vi "DDPoseEst2_DffDrive_Exec.vi"(8 "error in (no error)":errorcluster) -> (0 "error out":errorcluster)   [LabVIEW 2019]
uses:
  <vilib>/Rock Robotics/WPI/ThirdParty/JAS_Junk/TrajLib/Enum/DIFF_DRIVE_KitBot_WheelSize_ENUM.ctl
  <vilib>/Rock Robotics/WPI/ThirdParty/JAS_Junk/TrajLib/Enum/DIFF_DRIVE_ToughBoxMini_GearChoice_ENUM.ctl
  <vilib>/Rock Robotics/WPI/ThirdParty/JAS_Junk/TrajLib/Enum/DCMOTOR_TYPES_ENUM.ctl
  <vilib>/Rock Robotics/WPI/ThirdParty/JAS_Junk/TrajLib/LinearSystemId_CreateDriveTrainVelocitySystem.vi
  <vilib>/Rock Robotics/WPI/ThirdParty/JAS_Junk/TrajLib/DCMotor_PickMotor.vi
  <vilib>/Rock Robotics/WPI/ThirdParty/JAS_Junk/TrajLib/VI/numCmd_ObtainQueue_TwoDbl.vi
  <vilib>/Rock Robotics/WPI/ThirdParty/JAS_Junk/TrajLib/Units_InchesToMeters.vi
  <vilib>/Rock Robotics/WPI/ThirdParty/JAS_Junk/TrajLib/LinearSystem_New.vi
  <vilib>/Rock Robotics/WPI/ThirdParty/JAS_Junk/TrajLib/MatBuilder_Create.vi
  <vilib>/Rock Robotics/WPI/ThirdParty/JAS_Junk/TrajLib/MatBuilder_Fill.vi
  <vilib>/Rock Robotics/WPI/ThirdParty/JAS_Junk/TrajLib/MatrixHelper_Zero.vi
  <vilib>/Rock Robotics/WPI/ThirdParty/JAS_Junk/TrajLib/DCMotor_GetCIM.vi
  <vilib>/Rock Robotics/WPI/ThirdParty/JAS_Junk/TrajLib/DCMotor_GetAndymark9015.vi
  <vilib>/Rock Robotics/WPI/ThirdParty/JAS_Junk/TrajLib/DCMotor_GetAndymarkRs775_125.vi
  <vilib>/Rock Robotics/WPI/ThirdParty/JAS_Junk/TrajLib/DCMotor_GetBag.vi
  <vilib>/Rock Robotics/WPI/ThirdParty/JAS_Junk/TrajLib/DCMotor_GetBanebotsRs550.vi
  <vilib>/Rock Robotics/WPI/ThirdParty/JAS_Junk/TrajLib/DCMotor_GetBanebotsRs775.vi
  <vilib>/Rock Robotics/WPI/ThirdParty/JAS_Junk/TrajLib/DCMotor_GetFalcon500.vi
  <vilib>/Rock Robotics/WPI/ThirdParty/JAS_Junk/TrajLib/DCMotor_GetMiniCIM.vi
  <vilib>/Rock Robotics/WPI/ThirdParty/JAS_Junk/TrajLib/DCMotor_GetNEO.vi
  <vilib>/Rock Robotics/WPI/ThirdParty/JAS_Junk/TrajLib/DCMotor_GetNEO550.vi
  <vilib>/Rock Robotics/WPI/ThirdParty/JAS_Junk/TrajLib/DCMotor_GetRomiBuiltIn.vi
  <vilib>/Rock Robotics/WPI/ThirdParty/JAS_Junk/TrajLib/DCMotor_GetVex775Pro.vi
  <vilib>/Rock Robotics/WPI/ThirdParty/JAS_Junk/TrajLib/VI/DCMotor_GetAndymarkAM2235A.vi
  <vilib>/Rock Robotics/WPI/ThirdParty/JAS_Junk/TrajLib/VI/DCMotor_GetAndymarkAM3493.vi
  <vilib>/Rock Robotics/WPI/ThirdParty/JAS_Junk/TrajLib/Conv_Inches_Meters.vi
  <vilib>/Rock Robotics/WPI/ThirdParty/JAS_Junk/TrajLib/MatrixHelper_CoerceSize.vi
  <vilib>/Rock Robotics/WPI/ThirdParty/JAS_Junk/TrajLib/DCMotor_New.vi
  <vilib>/Rock Robotics/WPI/ThirdParty/JAS_Junk/TrajLib/VI/Units_RotationsPerMinuteToRadiansPerSecond.vi
  <vilib>/Rock Robotics/WPI/ThirdParty/JAS_Junk/TrajLib/Trajectory_Library.lvlib
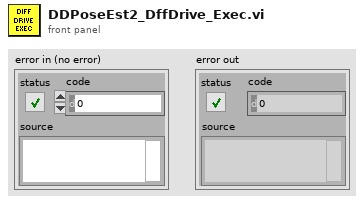
[diagram p1: front panel]
types:
  T1 = typedef "Trajectory_Library.lvlib/DIFF_DRIVE_KitBot_WheelSize_ENUM.ctl" = enum16{"4 Inch", "6 Inch", "8 Inch", "10 Inch"}
  T2 = typedef "Trajectory_Library.lvlib/DIFF_DRIVE_ToughBoxMini_GearChoice_ENUM.ctl" = enum16{"Ratio_12_75", "Ratio_10_71", "Ratio_8_45", "Ratio_7_31", "Ratio_5_95"}
  T3 = typedef "Trajectory_Library.lvlib/DCMOTOR_TYPES_ENUM.ctl" = enum16{"CIM", "AndyMark 9015", "Andy Mark RS 775 125", "Bag", "BaneBots RS 550", "BaneBots RS 775", "Falcon 500", "Mini CIM", "NEO", "NEO 550", "Romi BuiltIn", "Vex 775 Pro", "Snow Blower AM 2235A", "Bosch Seat AM 3493"}
  T4 = typedef "Trajectory_Library.lvlib/LINEAR_SYSTEM.ctl" = cluster{"m_A":T5, "m_B":T5, "m_C":T5, "m_D":T5, "States":i32, "Inputs":i32, "Outputs":i32}
  T5 = typedef "NI_Matrix.lvlib/RealMatrix.ctl" = dbl[][]
  T6 = typedef "Trajectory_Library.lvlib/LINEAR_SYSTEM_LOOP_DIFF_DRV_CTRL_PARAMS.CTL" = cluster{"Left Vel Model Std Dev m/s":dbl, "Left Vel Meas Std Dev m/s":dbl, "Left Vel Ctrl Tol m/s":dbl, "Max Control Effort":dbl, "Right Vel Ctrl Tol m/s":dbl, "Right Vel Meas Std Dev m/s":dbl, "Right Vel Model Std Dev m/s":dbl}
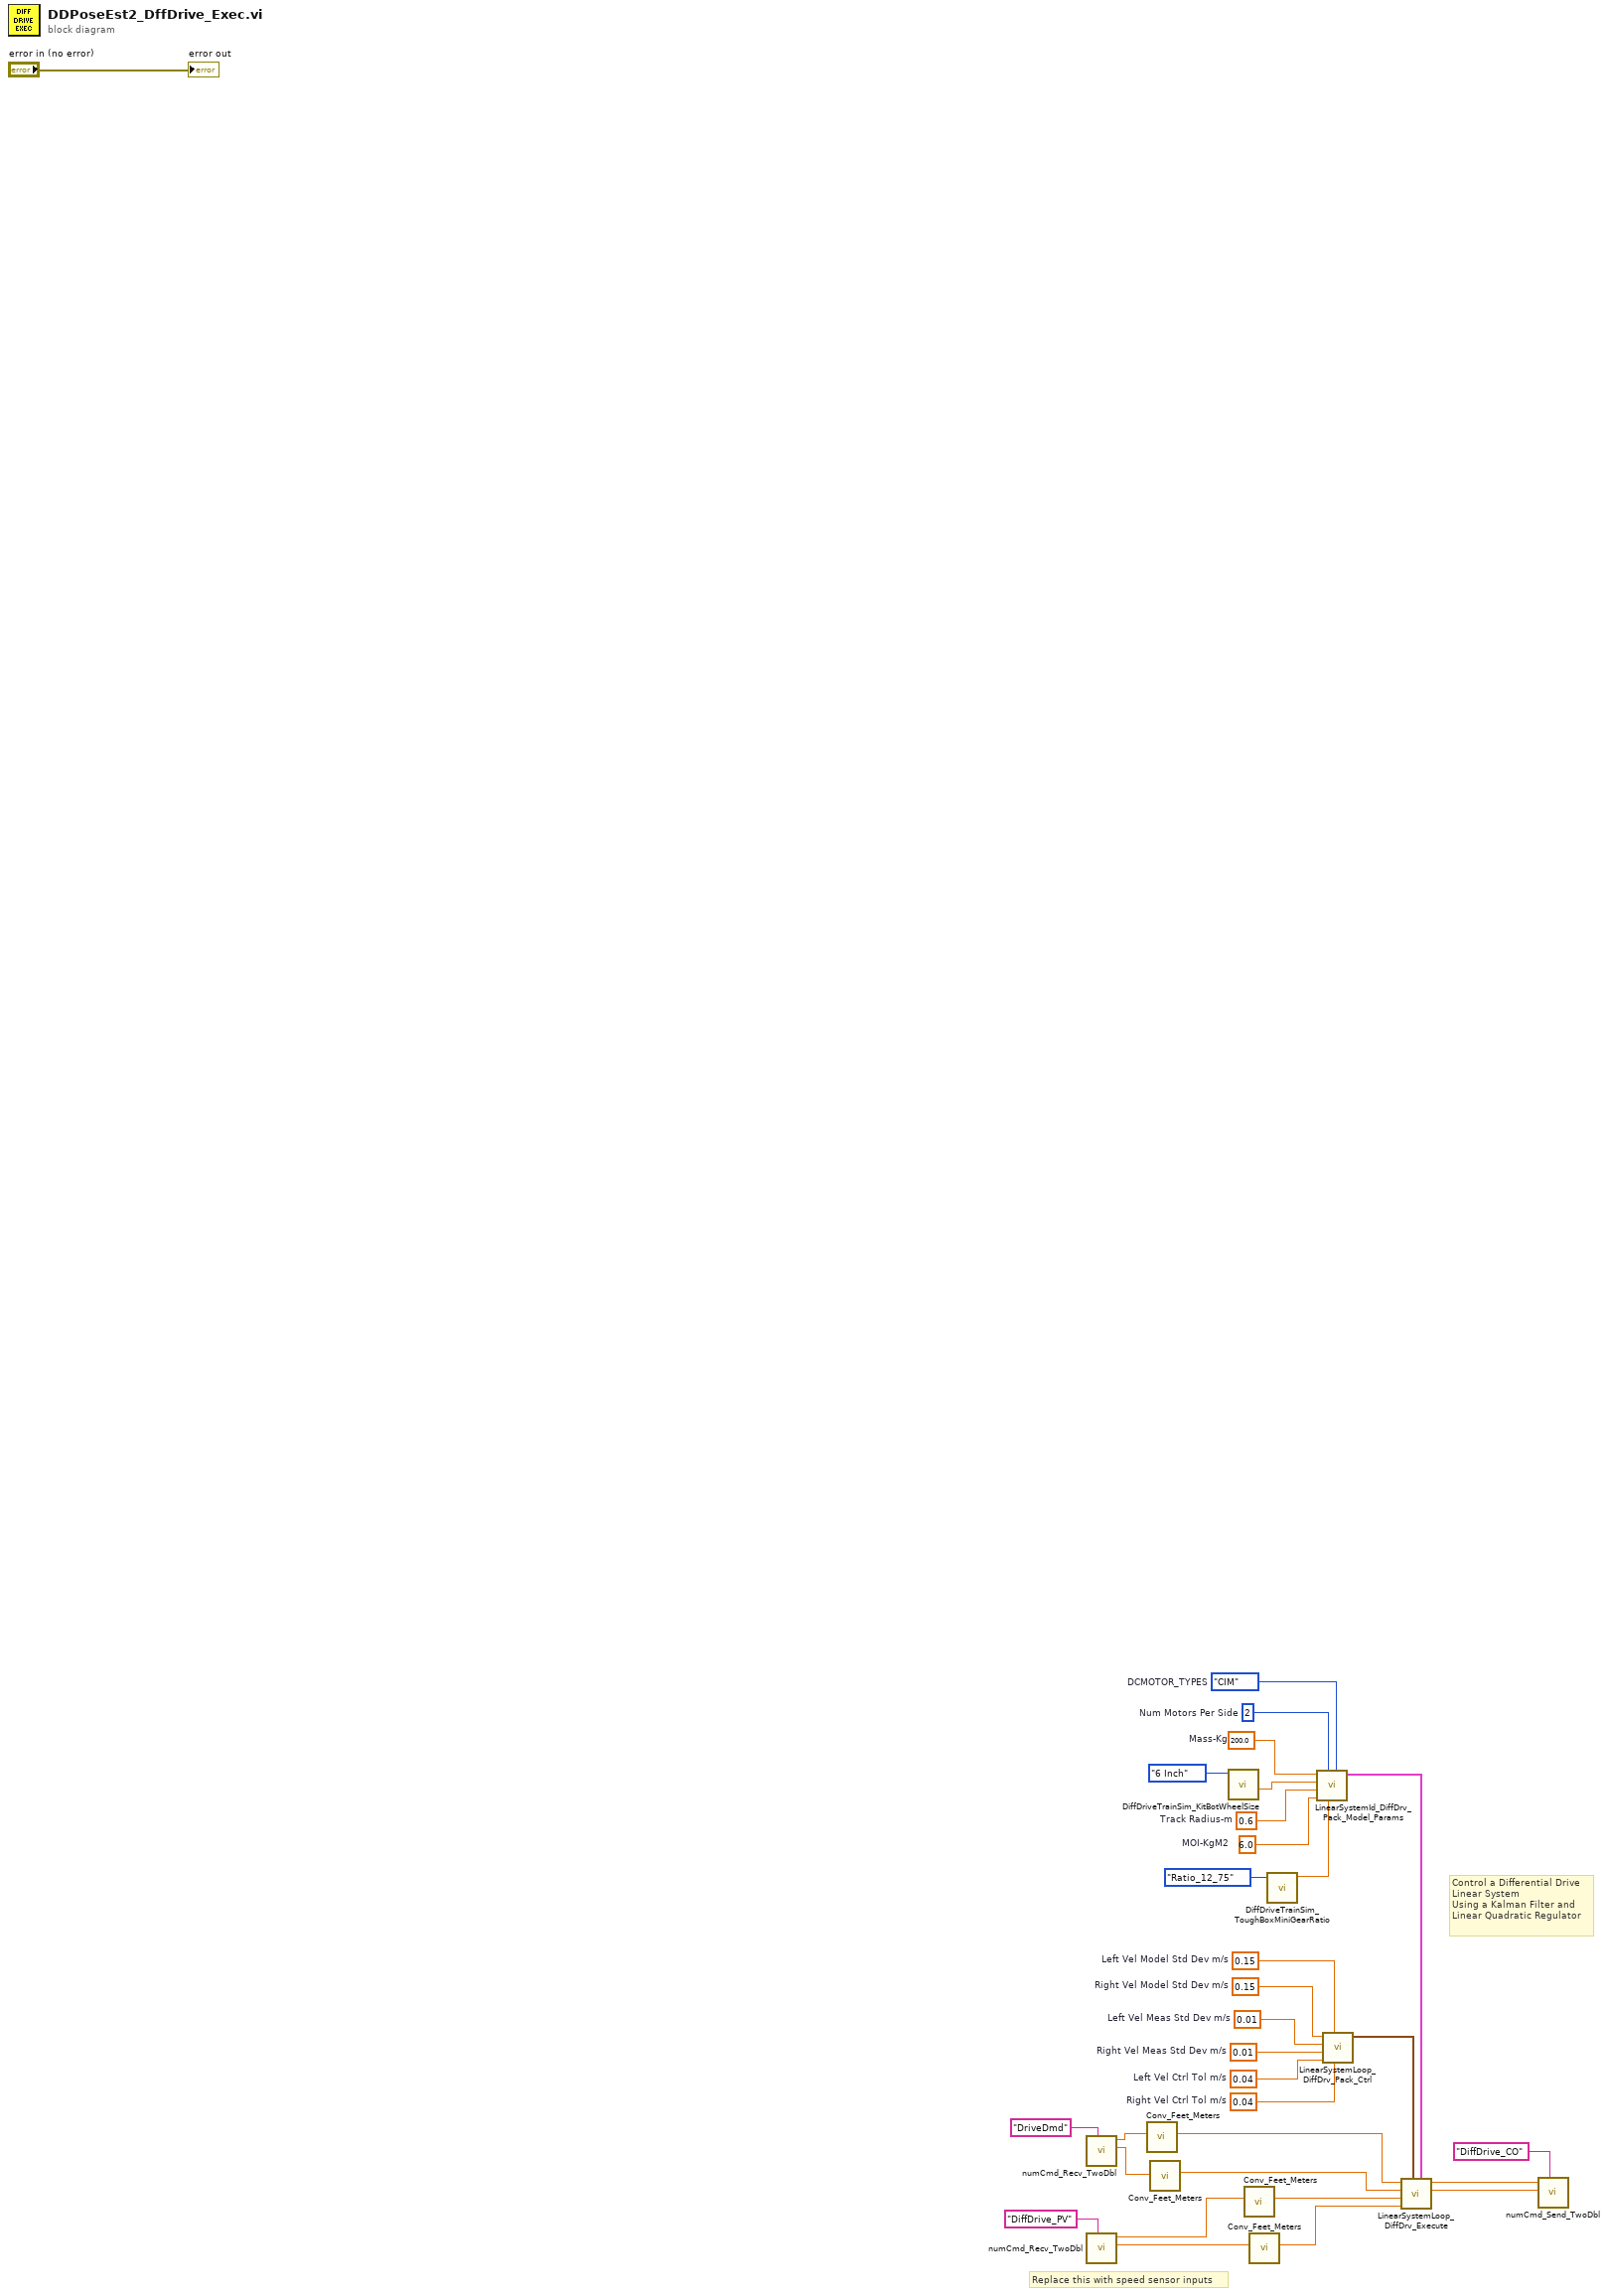
[diagram p0: block diagram]
diagram:
  w14 = 0.15  # Right Vel Model Std Dev m/s
  w13 = 0.01  # Left Vel Meas Std Dev m/s
  w12 = 0.01  # Right Vel Meas Std Dev m/s
  w11 = 0.04  # Left Vel Ctrl Tol m/s
  w10 = 0.15  # Left Vel Model Std Dev m/s
  w9 = 0.04  # Right Vel Ctrl Tol m/s
  w8 = 200.0  # Mass-Kg
  w7 = 0.6  # Track Radius-m
  w6 = 6.0  # MOI-KgM2
  w5 = 2  # Num Motors Per Side
  w4 = DCMOTOR_TYPES_ENUM."CIM"  # DCMOTOR_TYPES
  # "Replace this with speed sensor inputs"
  # "Control a Differential Drive\nLinear System\nUsing a Kalman Filter and \nLinear Quadratic Regulator"
  n1 = call <vilib>:"numCmd_Recv_TwoDbl.vi"("Command Name"="DriveDmd") -> ("Value 2"=w19:dbl, "Value 1"=w18:dbl)  [unwired: 7 in, 2 out]
  n2 = call <vilib>:"numCmd_Recv_TwoDbl.vi"("Command Name"="DiffDrive_PV") -> ("Value 2"=w24:dbl, "Value 1"=w23:dbl)  [unwired: 7 in, 2 out]
  n3 = call <vilib>:"Conv_Feet_Meters.vi"("Feet"=w18) -> ("Meters"=w15:dbl)  [unwired: 10 in]
  n4 = call <vilib>:"Conv_Feet_Meters.vi"("Feet"=w19) -> ("Meters"=w16:dbl)  [unwired: 10 in]
  n5 = call <vilib>:"DiffDriveTrainSim_KitBotWheelSize.vi"("Wheel Size"=DIFF_DRIVE_KitBot_WheelSize_ENUM."6 Inch") -> ("WheelRadius_M"=w31:dbl)  [unwired: 9 in, 1 out]
  n6 = call <vilib>:"Conv_Feet_Meters.vi"("Feet"=w23) -> ("Meters"=w20:dbl)  [unwired: 10 in]
  n7 = call <vilib>:"Conv_Feet_Meters.vi"("Feet"=w24) -> ("Meters"=w21:dbl)  [unwired: 10 in]
  n8 = call <vilib>:"DiffDriveTrainSim_ToughBoxMiniGearRatio.vi"("ToughBoxMiniGear"=DIFF_DRIVE_ToughBoxMini_GearChoice_ENUM."Ratio_12_75") -> ("GearRatio"=w29:dbl)  [unwired: 10 in]
  n9 = call <vilib>:"LinearSystemId_DiffDrv_Pack_Model_Params.vi"("DCMOTOR_TYPES"=w4, "Gear Ratio"=w29, "Num Motors Per Side"=w5, "MOI-KgM2"=w6, "Track Radius-m"=w7, "Wheel Radius-M"=w31, "Mass-Kg"=w8) -> ("DiffDrv_LinearSystem"=w3:T4)  [unwired: 4 in]
  n10 = call <vilib>:"LinearSystemLoop_DiffDrv_Pack_Ctrl.vi"("Right Vel Ctrl Tol m/s"=w9, "Left Vel Model Std Dev m/s"=w10, "Left Vel Ctrl Tol m/s"=w11, "Right Vel Meas Std Dev m/s"=w12, "Left Vel Meas Std Dev m/s"=w13, "Right Vel Model Std Dev m/s"=w14) -> ("LinearSystemLoop_DiffDrv_Ctrl_Params"=w2:T6)  [unwired: 5 in]
  n11 = call <vilib>:"LinearSystemLoop_DiffDrv_Execute.vi"("Linear System"=w3, "LinearSystemLoop_DiffDrv_Control_Params"=w2, "Right Vel PV m/s"=w21, "Left Vel PV m/s"=w20, "Right Vel SP m/s"=w16, "Left Vel SP m/s"=w15) -> ("Right Motor Dmd"=w27:dbl, "Left Motor Dmd"=w26:dbl)  [unwired: 1 in, 3 out]
  n12 = call <vilib>:"numCmd_Send_TwoDbl.vi"("Command Name"="DiffDrive_CO", "Value 2"=w27, "Value 1"=w26) -> ()  [unwired: 8 in, 1 out]
  "error out" <- "error in (no error)"
